vi "Publish Update.vi"(8 "error in (no error)":errorcluster, 11 "DAQmxAO in":refnum<class "DAQmxAO.lvclass">) -> (0 "error out":errorcluster, 3 "DAQmxAO out":refnum<class "DAQmxAO.lvclass">)   [LabVIEW 2020, in "VolatusDAQ.lvlib" / "DAQmxAO.lvclass"]
uses:
  DAQmxAO.lvclass
  DAQmxAO.lvclass/DAQmxAO.ctl
  VolatusData/VolatusData.lvlib
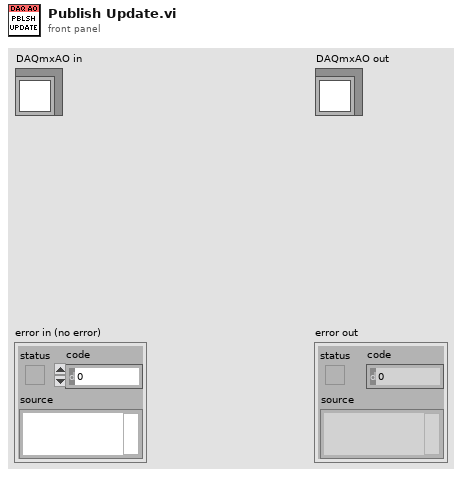
[diagram p1: front panel]
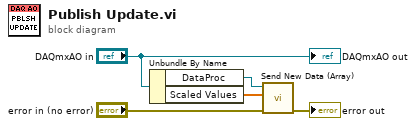
[diagram p0: block diagram]
diagram:
  n1 = Unbundle By Name("DAQmxAO in") -> ("DataProc"=w3:refnum<class "MessageQ.lvclass">, "Scaled Values"=w4:dbl[])
  n2 = call "Send New Data (Array).vi"("error in (no error)"="error in (no error)", "Data"=w4, "MessageQ"=w3) -> ("error out"=→"error out":errorcluster)  [unwired: 8 in]
  "DAQmxAO out" <- "DAQmxAO in"
